vi "Actor Core.vi"(8 "error in":errorcluster, 11 "Data Viewer in":refnum<class "Lissajous Viewer.lvclass">) -> (0 "error out":errorcluster, 3 "Actor out":refnum<class "Actor.lvclass">)   [LabVIEW 2020, in "Lissajous Viewer.lvlib" / "Lissajous Viewer.lvclass"]
doc: "The user interface for this panel.\n----\nCopyright: MGI 2016\nAuthor: Derek Trepanier"
uses:
  Lissajous Viewer.lvclass
  C:/Program Files/National Instruments/LabVIEW 2020/vi.lib/MGI/Panel Manager/Panel Actor/Panel Actor/Panel Actor.lvclass
  <vilib>/ActorFramework/Actor/Actor.lvclass
  Lissajous Viewer.lvclass/Lissajous Viewer.ctl
  <vilib>/MGI/Panel Manager/Panel Actor/Panel Actor/Panel Actor.lvclass
panel:
  in  "Wait indicator":bool
  out "Live Data":cluster{"Result":dbl[], "Result":dbl[]}(graph)
  out "Template Graph":cluster{"Result":dbl[], "Result":dbl[]}(graph)
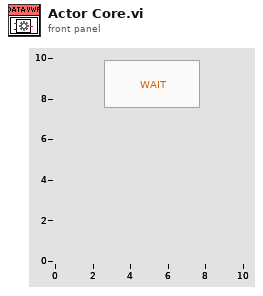
[diagram p1: front panel]
types:
  T1 = cluster{"Live Data":refnum<user-event>, "Template Data":refnum<user-event>, "Update Scaling":refnum<user-event>, "Acquire":refnum<user-event>}
  T2 = cluster{"Event Registration Refnum":refnum<event-registration>, "Pnl Actor":refnum<event-registration>}
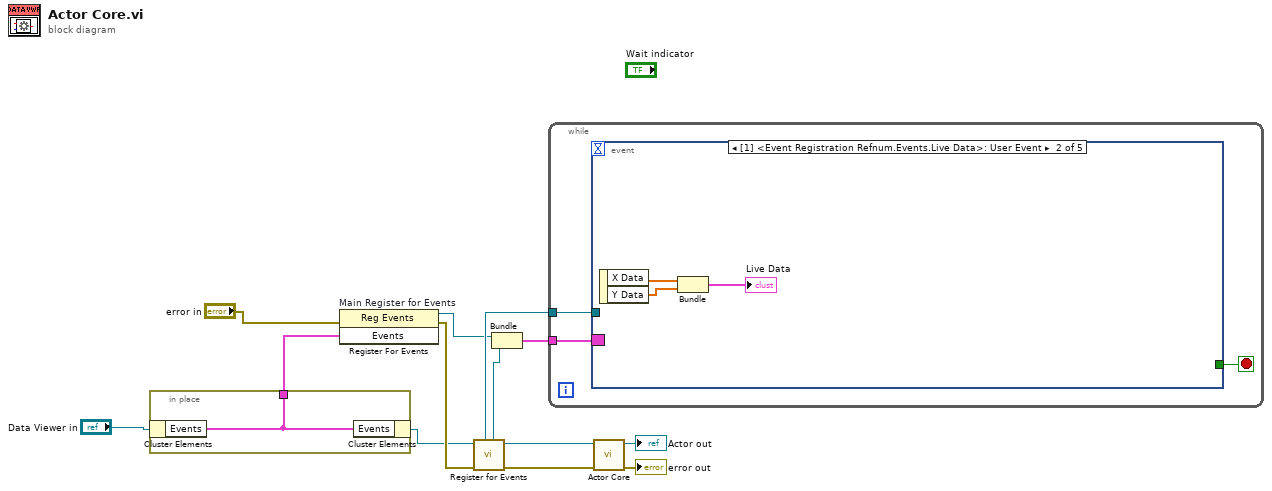
[diagram p0: block diagram]
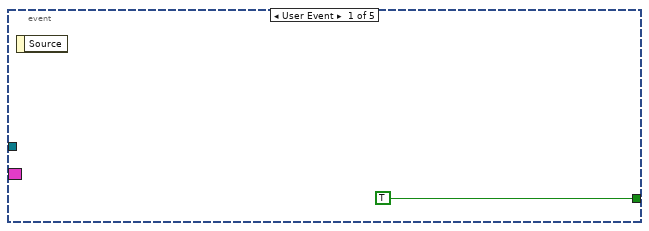
[diagram p2: hidden frame]
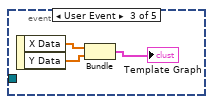
[diagram p3: hidden frame]
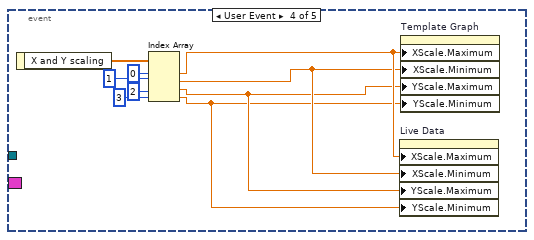
[diagram p4: hidden frame]
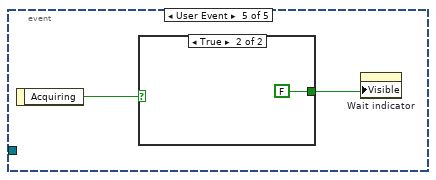
[diagram p5: hidden frame]
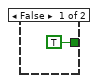
[diagram p6: hidden frame]
diagram:
  n1 = in-place {
    in-place-border: [w14] -> w7
    n2 = in-place-cluster #1("Data Viewer in") -> ("Events"=w14:T1)
    n3 = in-place-cluster #1("Events"=w14) -> (w1:refnum<class "Lissajous Viewer.lvclass">)
  }
  n4 = register-events "Main Register for Events"(error in="error in", w7) -> (reference out=w4:refnum<event-registration>, error out=w5:errorcluster)  [unwired: 1 in]
  n5 = call <vilib>:"Register for Events.vi"("Error In"=w5, "Panel Actor in"=w1) -> ("Error Out"=w11:errorcluster, "Panel Actor out"=w10:refnum<class "Lissajous Viewer.lvclass">, "Pnl Actor"=w3:refnum<event-registration>, "Self Enqueuer"=w9:refnum<class "Message Enqueuer.lvclass">)  [unwired: 6 in]
  n6 = Bundle("Event Registration Refnum"=w4, "Pnl Actor"=w3) -> (w2:T2)  [unwired: 1 in]
  n7 = while {
    tunnel: w2 -> [w17]
    tunnel: w9 -> [w15]
    stop <- w16 stop-if-true
    n8 = event shown="[1] <Event Registration Refnum.Events.Live Data>: User Event" {
      selector: w17 -> [_ _ _ _ _]
      dyn-events: _ -> [_ _ _ _ _]
      timeout: _ -> [_ _ _ _ _]
      tunnel: [TRUE _ _ _ _] -> w16
      tunnel: w15 -> [_ _ _ _ _]
      event User Event {
        n9 = event-data() -> ()  [unwired: 1 in, 1 out]
      }
      event User Event {
        n10 = event-data() -> ("X Data"=w21:dbl[], "Y Data"=w20:dbl[])  [unwired: 1 in]
        n11 = Bundle("X Data"=w21, "Y Data"=w20) -> (→"Live Data":cluster{"X Data":dbl[], "Y Data":dbl[]})  [unwired: 1 in]
      }
      event User Event {
        n12 = event-data() -> ("X Data"=w24:dbl[], "Y Data"=w23:dbl[])  [unwired: 1 in]
        n13 = Bundle("X Data"=w24, "Y Data"=w23) -> (→"Template Graph":cluster{"X Data":dbl[], "Y Data":dbl[]})  [unwired: 1 in]
      }
      event User Event {
        n14 = event-data() -> ("X and Y scaling"=w33:dbl[])  [unwired: 1 in]
        n15 = Index Array(array=w33, index #1=0 ("index"), index #2=1 ("index"), index #3=2 ("index"), index #4=3 ("index")) -> (element #1=w28:dbl, element #2=w27:dbl, element #3=w26:dbl, element #4=w25:dbl)
        n16 = property on="Live Data" class="XYGraph (strict)"("XScale.Maximum"=w28, "XScale.Minimum"=w27, "YScale.Maximum"=w26, "YScale.Minimum"=w25) -> ()  [unwired: 2 in, 2 out]
        n17 = property on="Template Graph" class="XYGraph (strict)"("XScale.Maximum"=w28, "XScale.Minimum"=w27, "YScale.Maximum"=w26, "YScale.Minimum"=w25) -> ()  [unwired: 2 in, 2 out]
      }
      event User Event {
        n18 = event-data() -> ("Acquiring"=w35:bool)  [unwired: 1 in]
        n19 = case shown="True" w35 {
          tunnel: [TRUE ("Visible") FALSE ("Visible")] -> w34
          frame False {
          }
          frame True {
          }
        }
        n20 = property on="Wait indicator" class="Bool"("Visible"=w34) -> ()  [unwired: 2 in, 2 out]
      }
    }
  }
  n21 = call-parent "Actor Core.vi"("error in"=w11, "Panel Actor in"=w10) -> ("error out"=→"error out":errorcluster, "Actor out"=→"Actor out":refnum<class "Actor.lvclass">)  [unwired: 8 in]
